vi "Set Unit.vi"(8 "error in (no error)":errorcluster, 11 "Keithley 622x2182 Driver in":refnum<class "Keithley 622x2182 Driver.lvclass">) -> (0 "error out":errorcluster, 3 "Keithley 622x2182 Driver out":refnum<class "Keithley 622x2182 Driver.lvclass">)   [LabVIEW 2021, in "Keithley 622x2182 Driver.lvclass"]
uses:
  Keithley 622x2182 Driver.lvclass
  C:/GitHub/NHMFL_Core/Libraries/Instruments/VISA Instrument/VISA Instrument.lvclass
  VISA Instrument/VISA Instrument.lvclass/VISA Instrument.ctl
  VISA Instrument/Read VISA resource.vi
  VISA Instrument/Write VISA resource.vi
  Keithley 622x2182 Driver.lvclass/Keithley 622x2182 Driver.ctl
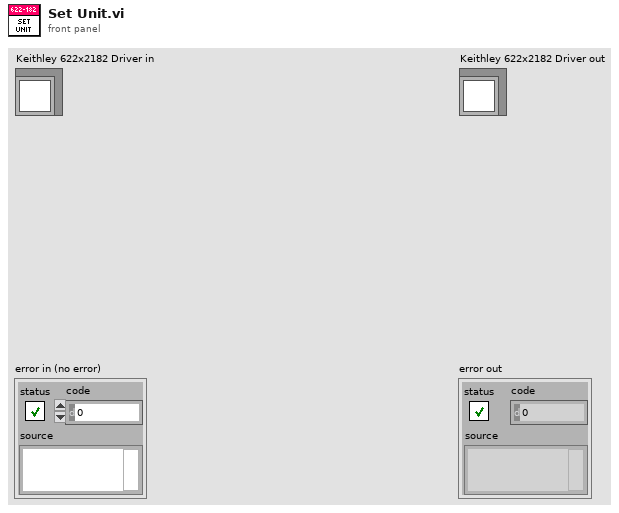
[diagram p1: front panel]
types:
  T1 = typedef "Unit.ctl" = enum16{"Volt", "Ohm", "Siemens"}
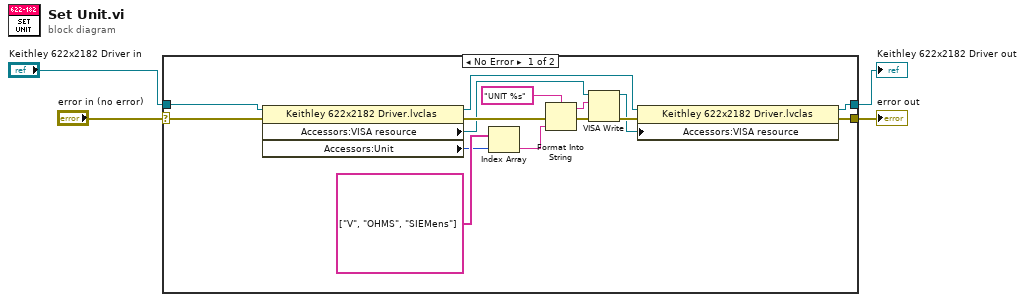
[diagram p0: block diagram]
diagram:
  n1 = case shown="No Error" "error in (no error)" {
    selector: "error in (no error)" -> [w6 w21]
    tunnel: [w5 w21] -> w3
    tunnel: [w13 w20] -> w1
    tunnel: "Keithley 622x2182 Driver in" -> [w11 w20]
    frame No Error {
      n2 = property class="Keithley 622x2182 Driver.lvclas"(reference=w11, error in=w6) -> (reference out=w12:refnum<class "Keithley 622x2182 Driver.lvclass">, error out=w15:errorcluster, "Accessors:VISA resource"=w8:refnum<visa-resource-name>, "Accessors:Unit"=w18:T1)
      n3 = Index Array(array=string[] ["V", "OHMS", "SIEMens"], index=w18) -> (element=w17:string)
      n4 = Format Into String(format string="UNIT %s", error in=w15, w17) -> (resulting string=w16:string, error out=w14:errorcluster)  [unwired: 1 in]
      n5 = VISA Write(VISA resource name=w8, write buffer=w16, error in (no error)=w14) -> (VISA resource name out=w9:refnum<visa-resource-name>, error out=w10:errorcluster)  [unwired: 1 out]
      n6 = property class="Keithley 622x2182 Driver.lvclas"(reference=w12, error in=w10, "Accessors:VISA resource"=w9) -> (reference out=w13:refnum<class "Keithley 622x2182 Driver.lvclass">, error out=w5:errorcluster)
    }
    frame Error {
    }
  }
  "error out" <- w3
  "Keithley 622x2182 Driver out" <- w1
